vi "L2 Offset Conversions.vi"(8 "error in (no error)":errorcluster, 10 "Inputs":dbl[](array[numeric]), 11 "ConversionOps":T1) -> (0 "error out":errorcluster, 2 "Outputs":dbl[](array[numeric]))   [LabVIEW 2013]
uses:
  Conversion Operations.ctl
  Data Access Objects/Metadata/Persistant DAO Actions.ctl
  Data Access Objects/Metadata/DAO Actions with Remove.ctl
  Data Access Objects/Metadata/LBCB Number.ctl
  LbcbConversionTypes.ctl
  C:/Users/mbletzin/Desktop/Work/NewLbcbConversionDll/DLL/LbcbConversions.dll
  DLL/LbcbConversions.dll
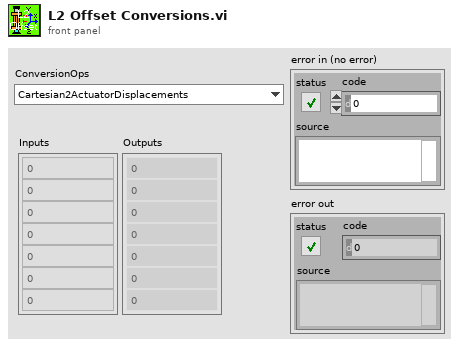
[diagram p1: front panel]
types:
  T1 = typedef "Conversion Operations.ctl" = enum16{"Cartesian2ActuatorDisplacements", "Actuator2CartesianDisplacements", "Actuators2CartesianForces", "Initialize"}
  T2 = typedef "Persistant DAO Actions.ctl" = enum16{"Init", "Get", "Set", "Load", "Save"}
  T3 = typedef "LbcbConversionTypes.ctl" = enum16{"Commands", "Readings", "Offsets"}
  T4 = typedef "LBCB Number.ctl" = enum16{"LBCB1", "LBCB2"}
  T5 = typedef "DAO Actions with Remove.ctl" = enum16{"Init", "Get", "Set", "Remove"}
  T6 = typedef "Number Of LBCBs.ctl" = enum16{"1", "2"}
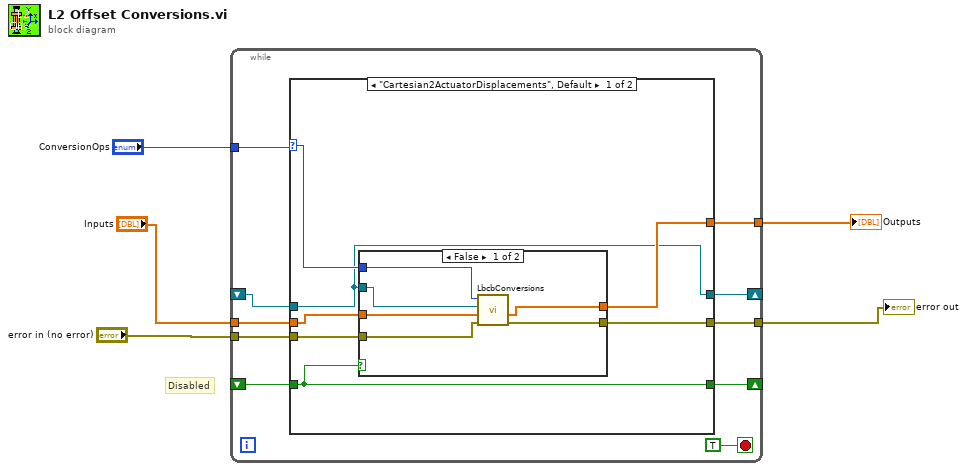
[diagram p0: block diagram]
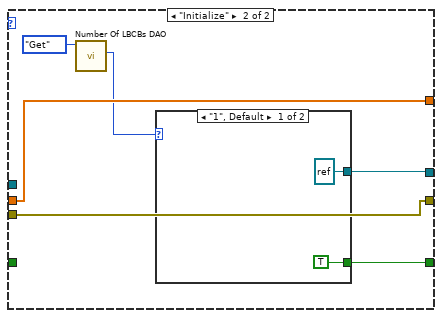
[diagram p3: hidden frame]
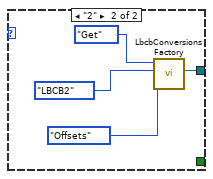
[diagram p4: hidden frame]
diagram:
  # "Disabled"
  n1 = while {
    tunnel: "ConversionOps" -> [w14]
    shift-right: [w13] -> _
    shift-left: _ -> [w12]
    tunnel: "Inputs" -> [w11]
    tunnel: [w10] -> w3
    tunnel: [w9] -> w2
    tunnel: "error in (no error)" -> [w8]
    shift-right: [w7] -> _
    shift-left: _ -> [w6]
    stop <- TRUE stop-if-true
    n2 = case shown="\"Cartesian2ActuatorDisplacements\", Default" w14 {
      selector: w14 -> [w22 _]
      tunnel: [w19 w36] -> w13
      tunnel: w12 -> [w19 _]
      tunnel: w11 -> [w21 w35]
      tunnel: [w20 w35] -> w10
      tunnel: [w18 w34] -> w9
      tunnel: w8 -> [w17 w34]
      tunnel: [w16 w31] -> w7
      tunnel: w6 -> [w16 _]
      frame "Cartesian2ActuatorDisplacements", Default {
        n3 = case shown="False" w16 {
          tunnel: w22 -> [w28 _]
          tunnel: w21 -> [w27 w30]
          tunnel: [w26 w30] -> w20
          tunnel: w19 -> [w25 _]
          tunnel: [w24 w29] -> w18
          tunnel: w17 -> [w23 w29]
          frame False {
            n4 = call "LbcbConversions.vi"("error in (no error)"=w23, "Inputs"=w27, "Conversion Ref"=w25, "ConversionOps"=w28) -> ("error out"=w24:errorcluster, "Outputs"=w26:dbl[])  [unwired: 6 in]
          }
          frame True {
          }
        }
      }
      frame "Initialize" {
        n5 = call "Number Of LBCBs DAO.vi"("Actions"=Persistant_DAO_Actions."Get") -> ("Number of\nLBCBs Out"=w32:T6)  [unwired: 7 in, 3 out]
        n6 = case shown="\"1\", Default" w32 {
          tunnel: [refnum<k24> refnum ("Conversion Ref") w42] -> w36
          tunnel: [TRUE _] -> w31
          frame "1", Default {
          }
          frame "2" {
            n7 = call "LbcbConversionsFactory.vi"("LbcbConversionType"=LbcbConversionTypes."Offsets", "LBCB Number"=LBCB_Number."LBCB2", "Actions"=DAO_Actions_with_Remove."Get") -> ("Conversion Ref"=w42:refnum<k24>)  [unwired: 7 in, 1 out]
          }
        }
      }
    }
  }
  "Outputs" <- w3
  "error out" <- w2
